vi "Peak Detector PtByPt.vi"(0 "x":dbl format="%0.2f", 1 "threshold peak":dbl format="%0.2f", 2 "threshold valley":dbl format="%0.2f", 3 "width":i32=3, 4 "initialize":bool) -> (5 "peak":bool, 6 "valley":bool, 7 "error":i32)   [LabVIEW 2017, in "NI_PtbyPt.lvlib"]
doc: "Finds the location of peaks or valleys in the set of input data points specified by <B>width</B>."
uses:
  <vilib>/ptbypt/NI_PtbyPt.lvlib
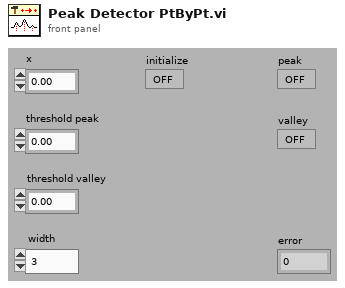
[diagram p1: front panel]
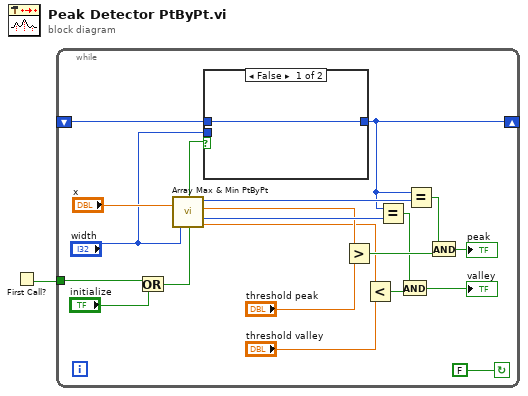
[diagram p0: block diagram]
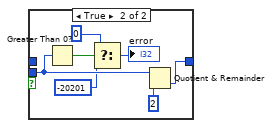
[diagram p2: hidden frame]
diagram:
  n1 = First Call?() -> (First Call?: T/F=w1:bool)
  n2 = while {
    tunnel: w1 -> [w4]
    shift-left: _ -> [w17]
    shift-right: [w16] -> _
    stop <- FALSE continue-if-true
    n3 = Or(x=w4, y="initialize") -> (x .or. y?=w2:bool)
    n4 = call <vilib>:"Array Max & Min PtByPt.vi"("input data point"="x", "sample length"="width", "initialize"=w2) -> ("max index"=w21:i32, "max value"=w11:dbl, "min index"=w15:i32, "min value"=w10:dbl)  [unwired: 1 out]
    n5 = case shown="False" w2 {
      tunnel: [w22 w28] -> w16
      tunnel: w17 -> [w22 _]
      tunnel: "width" -> [_ w27]
      frame False {
      }
      frame True {
        n6 = Greater Than 0?(x=w27) -> (x > 0?=w26:bool)
        n7 = Select(t=0, s=w26, f=-20201) -> (s? t:f=→"error":i32)
        n8 = Quotient & Remainder(x=w27, y=2) -> (floor(x/y)=w28:i32)  [unwired: 1 out]
      }
    }
    n9 = Greater?(x=w11, y="threshold peak") -> (0:w19:bool)
    n10 = Less?(x=w10, y="threshold valley") -> (x < y?=w13:bool)
    n11 = Equal?(x=w16, y=w15) -> (x = y?=w14:bool)
    n12 = And(x=w14, y=w13) -> (x .and. y?=→"valley":bool)
    n13 = Equal?(x=w16, y=w21) -> (x = y?=w20:bool)
    n14 = And(x=w20, y=w19) -> (x .and. y?=→"peak":bool)
  }
